vi "DDS_Clock.vi"() -> ()   [LabVIEW 2016] (continued)
  out "frequency-time plot":T6(graph)=[{[{"total time[ms]"=0.0, "f1 [Hz] CH0"=300000000.0}, {"total time[ms]"=0.05, "f1 [Hz] CH0"=300200000.0}, {"total time[ms]"=0.05, "f1 [Hz] CH0"=300200000.0}, {"total time[ms]"=0.1, "f1 [Hz] CH0"=300400000.0}, {"total time[ms]"=0.1, "f1 [Hz] CH0"=300400000.0}, {"total time[ms]"=0.15000000000000002, "f1 [Hz] CH0"=300600000.0}, {"total time[ms]"=0.15000000000000002, "f1 [Hz] CH0"=300600000.0}, {"total time[ms]"=0.2, "f1 [Hz] CH0"=300800000.0}, {"total time[ms]"=0.2, "f1 [Hz] CH0"=300800000.0}, {"total time[ms]"=0.25, "f1 [Hz] CH0"=301000000.0}, {"total time[ms]"=0.25, "f1 [Hz] CH0"=301000000.0}, {"total time[ms]"=0.3, "f1 [Hz] CH0"=301200000.0}, {"total time[ms]"=0.3, "f1 [Hz] CH0"=301200000.0}, {"total time[ms]"=0.35, "f1 [Hz] CH0"=301400000.0}, {"total time[ms]"=0.35, "f1 [Hz] CH0"=301400000.0}, {"total time[ms]"=0.39999999999999997, "f1 [Hz] CH0"=301600000.0}, {"total time[ms]"=0.39999999999999997, "f1 [Hz] CH0"=301600000.0}, {"total time[ms]"=0.44999999999999996, "f1 [Hz] CH0"=301800000.0}, {"total time[ms]"=0.44999999999999996, "f1 [Hz] CH0"=301800000.0}, {"total time[ms]"=0.49999999999999994, "f1 [Hz] CH0"=302000000.0}, {"total time[ms]"=0.49999999999999994, "f1 [Hz] CH0"=302000000.0}, {"total time[ms]"=0.5499999999999999, "f1 [Hz] CH0"=302200000.0}, {"total time[ms]"=0.5499999999999999, "f1 [Hz] CH0"=302200000.0}, {"total time[ms]"=0.6, "f1 [Hz] CH0"=302400000.0}, {"total time[ms]"=0.6, "f1 [Hz] CH0"=302400000.0}, {"total time[ms]"=0.65, "f1 [Hz] CH0"=302600000.0}, {"total time[ms]"=0.65, "f1 [Hz] CH0"=302600000.0}, {"total time[ms]"=0.7000000000000001, "f1 [Hz] CH0"=302800000.0}, {"total time[ms]"=0.7000000000000001, "f1 [Hz] CH0"=302800000.0}, {"total time[ms]"=0.7500000000000001, "f1 [Hz] CH0"=303000000.0}, {"total time[ms]"=0.7500000000000001, "f1 [Hz] CH0"=303000000.0}, {"total time[ms]"=0.8000000000000002, "f1 [Hz] CH0"=303200000.0}, {"total time[ms]"=0.8000000000000002, "f1 [Hz] CH0"=303200000.0}, {"total time[ms]"=0.8500000000000002, "f1 [Hz] CH0"=303400000.0}, {"total time[ms]"=0.8500000000000002, "f1 [Hz] CH0"=303400000.0}, {"total time[ms]"=0.9000000000000002, "f1 [Hz] CH0"=303600000.0}, {"total time[ms]"=0.9000000000000002, "f1 [Hz] CH0"=303600000.0}, {"total time[ms]"=0.9500000000000003, "f1 [Hz] CH0"=303800000.0}, {"total time[ms]"=0.9500000000000003, "f1 [Hz] CH0"=303800000.0}, {"total time[ms]"=1.0000000000000002, "f1 [Hz] CH0"=304000000.0}, {"total time[ms]"=1.0000000000000002, "f1 [Hz] CH0"=304000000.0}, {"total time[ms]"=1.0500000000000003, "f1 [Hz] CH0"=304200000.0}, {"total time[ms]"=1.0500000000000003, "f1 [Hz] CH0"=304200000.0}, {"total time[ms]"=1.1000000000000003, "f1 [Hz] CH0"=304400000.0}, {"total time[ms]"=1.1000000000000003, "f1 [Hz] CH0"=304400000.0}, {"total time[ms]"=1.1500000000000004, "f1 [Hz] CH0"=304600000.0}, {"total time[ms]"=1.1500000000000004, "f1 [Hz] CH0"=304600000.0}, {"total time[ms]"=1.2000000000000004, "f1 [Hz] CH0"=304800000.0}, {"total time[ms]"=1.2000000000000004, "f1 [Hz] CH0"=304800000.0}, {"total time[ms]"=1.2500000000000004, "f1 [Hz] CH0"=305000000.0}, {"total time[ms]"=1.2500000000000004, "f1 [Hz] CH0"=305000000.0}, {"total time[ms]"=1.3000000000000005, "f1 [Hz] CH0"=305200000.0}, {"total time[ms]"=1.3000000000000005, "f1 [Hz] CH0"=305200000.0}, {"total time[ms]"=1.3500000000000005, "f1 [Hz] CH0"=305400000.0}, {"total time[ms]"=1.3500000000000005, "f1 [Hz] CH0"=305400000.0}, {"total time[ms]"=1.4000000000000006, "f1 [Hz] CH0"=305600000.0}, {"total time[ms]"=1.4000000000000006, "f1 [Hz] CH0"=305600000.0}, {"total time[ms]"=1.4500000000000006, "f1 [Hz] CH0"=305800000.0}, {"total time[ms]"=1.4500000000000006, "f1 [Hz] CH0"=305800000.0}, {"total time[ms]"=1.5000000000000007, "f1 [Hz] CH0"=306000000.0}, {"total time[ms]"=1.5000000000000007, "f1 [Hz] CH0"=306000000.0}, {"total time[ms]"=1.5500000000000007, "f1 [Hz] CH0"=306200000.0}, {"total time[ms]"=1.5500000000000007, "f1 [Hz] CH0"=306200000.0}, {"total time[ms]"=1.6000000000000008, "f1 [Hz] CH0"=306400000.0}, {"total time[ms]"=1.6000000000000008, "f1 [Hz] CH0"=306400000.0}, {"total time[ms]"=1.6500000000000008, "f1 [Hz] CH0"=306600000.0}, {"total time[ms]"=1.6500000000000008, "f1 [Hz] CH0"=306600000.0}, {"total time[ms]"=1.7000000000000008, "f1 [Hz] CH0"=306800000.0}, {"total time[ms]"=1.7000000000000008, "f1 [Hz] CH0"=306800000.0}, {"total time[ms]"=1.7500000000000009, "f1 [Hz] CH0"=307000000.0}, {"total time[ms]"=1.7500000000000009, "f1 [Hz] CH0"=307000000.0}, {"total time[ms]"=1.800000000000001, "f1 [Hz] CH0"=307200000.0}, {"total time[ms]"=1.800000000000001, "f1 [Hz] CH0"=307200000.0}, {"total time[ms]"=1.850000000000001, "f1 [Hz] CH0"=307400000.0}, {"total time[ms]"=1.850000000000001, "f1 [Hz] CH0"=307400000.0}, {"total time[ms]"=1.900000000000001, "f1 [Hz] CH0"=307600000.0}, {"total time[ms]"=1.900000000000001, "f1 [Hz] CH0"=307600000.0}, {"total time[ms]"=1.950000000000001, "f1 [Hz] CH0"=307800000.0}, {"total time[ms]"=1.950000000000001, "f1 [Hz] CH0"=307800000.0}, {"total time[ms]"=2.000000000000001, "f1 [Hz] CH0"=308000000.0}, {"total time[ms]"=2.000000000000001, "f1 [Hz] CH0"=308000000.0}, {"total time[ms]"=2.0500000000000007, "f1 [Hz] CH0"=308200000.0}, {"total time[ms]"=2.0500000000000007, "f1 [Hz] CH0"=308200000.0}, {"total time[ms]"=2.1000000000000005, "f1 [Hz] CH0"=308400000.0}, {"total time[ms]"=2.1000000000000005, "f1 [Hz] CH0"=308400000.0}, {"total time[ms]"=2.1500000000000004, "f1 [Hz] CH0"=308600000.0}, {"total time[ms]"=2.1500000000000004, "f1 [Hz] CH0"=308600000.0}, {"total time[ms]"=2.2, "f1 [Hz] CH0"=308800000.0}, {"total time[ms]"=2.2, "f1 [Hz] CH0"=308800000.0}, {"total time[ms]"=2.25, "f1 [Hz] CH0"=309000000.0}, {"total time[ms]"=2.25, "f1 [Hz] CH0"=309000000.0}, {"total time[ms]"=2.3, "f1 [Hz] CH0"=309200000.0}, {"total time[ms]"=2.3, "f1 [Hz] CH0"=309200000.0}, {"total time[ms]"=2.3499999999999996, "f1 [Hz] CH0"=309400000.0}, {"total time[ms]"=2.3499999999999996, "f1 [Hz] CH0"=309400000.0}, {"total time[ms]"=2.3999999999999995, "f1 [Hz] CH0"=309600000.0}, {"total time[ms]"=2.3999999999999995, "f1 [Hz] CH0"=309600000.0}, {"total time[ms]"=2.4499999999999993, "f1 [Hz] CH0"=309800000.0}, {"total time[ms]"=2.4499999999999993, "f1 [Hz] CH0"=309800000.0}, {"total time[ms]"=2.499999999999999, "f1 [Hz] CH0"=310000000.0}, {"total time[ms]"=2.499999999999999, "f1 [Hz] CH0"=310000000.0}, {"total time[ms]"=2.549999999999999, "f1 [Hz] CH0"=310200000.0}, {"total time[ms]"=2.549999999999999, "f1 [Hz] CH0"=310200000.0}, {"total time[ms]"=2.5999999999999988, "f1 [Hz] CH0"=310400000.0}, {"total time[ms]"=2.5999999999999988, "f1 [Hz] CH0"=310400000.0}, {"total time[ms]"=2.6499999999999986, "f1 [Hz] CH0"=310600000.0}, {"total time[ms]"=2.6499999999999986, "f1 [Hz] CH0"=310600000.0}, {"total time[ms]"=2.6999999999999984, "f1 [Hz] CH0"=310800000.0}, {"total time[ms]"=2.6999999999999984, "f1 [Hz] CH0"=310800000.0}, {"total time[ms]"=2.7499999999999982, "f1 [Hz] CH0"=311000000.0}, {"total time[ms]"=2.7499999999999982, "f1 [Hz] CH0"=311000000.0}, {"total time[ms]"=2.799999999999998, "f1 [Hz] CH0"=311200000.0}, {"total time[ms]"=2.799999999999998, "f1 [Hz] CH0"=311200000.0}, {"total time[ms]"=2.849999999999998, "f1 [Hz] CH0"=311400000.0}, {"total time[ms]"=2.849999999999998, "f1 [Hz] CH0"=311400000.0}, {"total time[ms]"=2.8999999999999977, "f1 [Hz] CH0"=311600000.0}, {"total time[ms]"=2.8999999999999977, "f1 [Hz] CH0"=311600000.0}, {"total time[ms]"=2.9499999999999975, "f1 [Hz] CH0"=311800000.0}, {"total time[ms]"=2.9499999999999975, "f1 [Hz] CH0"=311800000.0}, {"total time[ms]"=2.9999999999999973, "f1 [Hz] CH0"=312000000.0}, {"total time[ms]"=2.9999999999999973, "f1 [Hz] CH0"=312000000.0}, {"total time[ms]"=3.049999999999997, "f1 [Hz] CH0"=312200000.0}, {"total time[ms]"=3.049999999999997, "f1 [Hz] CH0"=312200000.0}, {"total time[ms]"=3.099999999999997, "f1 [Hz] CH0"=312400000.0}, {"total time[ms]"=3.099999999999997, "f1 [Hz] CH0"=312400000.0}, {"total time[ms]"=3.149999999999997, "f1 [Hz] CH0"=312600000.0}, {"total time[ms]"=3.149999999999997, "f1 [Hz] CH0"=312600000.0}, {"total time[ms]"=3.1999999999999966, "f1 [Hz] CH0"=312800000.0}, {"total time[ms]"=3.1999999999999966, "f1 [Hz] CH0"=312800000.0}, {"total time[ms]"=3.2499999999999964, "f1 [Hz] CH0"=313000000.0}, {"total time[ms]"=3.2499999999999964, "f1 [Hz] CH0"=313000000.0}, {"total time[ms]"=3.2999999999999963, "f1 [Hz] CH0"=313200000.0}, {"total time[ms]"=3.2999999999999963, "f1 [Hz] CH0"=313200000.0}, {"total time[ms]"=3.349999999999996, "f1 [Hz] CH0"=313400000.0}, {"total time[ms]"=3.349999999999996, "f1 [Hz] CH0"=313400000.0}, {"total time[ms]"=3.399999999999996, "f1 [Hz] CH0"=313600000.0}, {"total time[ms]"=3.399999999999996, "f1 [Hz] CH0"=313600000.0}, {"total time[ms]"=3.4499999999999957, "f1 [Hz] CH0"=313800000.0}, {"total time[ms]"=3.4499999999999957, "f1 [Hz] CH0"=313800000.0}, {"total time[ms]"=3.4999999999999956, "f1 [Hz] CH0"=314000000.0}, {"total time[ms]"=3.4999999999999956, "f1 [Hz] CH0"=314000000.0}, {"total time[ms]"=3.5499999999999954, "f1 [Hz] CH0"=314200000.0}, {"total time[ms]"=3.5499999999999954, "f1 [Hz] CH0"=314200000.0}, {"total time[ms]"=3.599999999999995, "f1 [Hz] CH0"=314400000.0}, {"total time[ms]"=3.599999999999995, "f1 [Hz] CH0"=314400000.0}, {"total time[ms]"=3.649999999999995, "f1 [Hz] CH0"=314600000.0}, {"total time[ms]"=3.649999999999995, "f1 [Hz] CH0"=314600000.0}, {"total time[ms]"=3.699999999999995, "f1 [Hz] CH0"=314800000.0}, {"total time[ms]"=3.699999999999995, "f1 [Hz] CH0"=314800000.0}, {"total time[ms]"=3.7499999999999947, "f1 [Hz] CH0"=315000000.0}, {"total time[ms]"=3.7499999999999947, "f1 [Hz] CH0"=315000000.0}, {"total time[ms]"=3.7999999999999945, "f1 [Hz] CH0"=315200000.0}, {"total time[ms]"=3.7999999999999945, "f1 [Hz] CH0"=315200000.0}, {"total time[ms]"=3.8499999999999943, "f1 [Hz] CH0"=315400000.0}, {"total time[ms]"=3.8499999999999943, "f1 [Hz] CH0"=315400000.0}, {"total time[ms]"=3.899999999999994, "f1 [Hz] CH0"=315600000.0}, {"total time[ms]"=3.899999999999994, "f1 [Hz] CH0"=315600000.0}, {"total time[ms]"=3.949999999999994, "f1 [Hz] CH0"=315800000.0}, {"total time[ms]"=3.949999999999994, "f1 [Hz] CH0"=315800000.0}, {"total time[ms]"=3.999999999999994, "f1 [Hz] CH0"=316000000.0}, {"total time[ms]"=3.999999999999994, "f1 [Hz] CH0"=316000000.0}, {"total time[ms]"=4.049999999999994, "f1 [Hz] CH0"=316200000.0}, {"total time[ms]"=4.049999999999994, "f1 [Hz] CH0"=316200000.0}, {"total time[ms]"=4.099999999999993, "f1 [Hz] CH0"=316400000.0}, {"total time[ms]"=4.099999999999993, "f1 [Hz] CH0"=316400000.0}, {"total time[ms]"=4.149999999999993, "f1 [Hz] CH0"=316600000.0}, {"total time[ms]"=4.149999999999993, "f1 [Hz] CH0"=316600000.0}, {"total time[ms]"=4.199999999999993, "f1 [Hz] CH0"=316800000.0}, {"total time[ms]"=4.199999999999993, "f1 [Hz] CH0"=316800000.0}, {"total time[ms]"=4.249999999999993, "f1 [Hz] CH0"=317000000.0}, {"total time[ms]"=4.249999999999993, "f1 [Hz] CH0"=317000000.0}, {"total time[ms]"=4.299999999999993, "f1 [Hz] CH0"=317200000.0}, {"total time[ms]"=4.299999999999993, "f1 [Hz] CH0"=317200000.0}, {"total time[ms]"=4.3499999999999925, "f1 [Hz] CH0"=317400000.0}, {"total time[ms]"=4.3499999999999925, "f1 [Hz] CH0"=317400000.0}, {"total time[ms]"=4.399999999999992, "f1 [Hz] CH0"=317600000.0}, {"total time[ms]"=4.399999999999992, "f1 [Hz] CH0"=317600000.0}, {"total time[ms]"=4.449999999999992, "f1 [Hz] CH0"=317800000.0}, {"total time[ms]"=4.449999999999992, "f1 [Hz] CH0"=317800000.0}, {"total time[ms]"=4.499999999999992, "f1 [Hz] CH0"=318000000.0}, {"total time[ms]"=4.499999999999992, "f1 [Hz] CH0"=318000000.0}, {"total time[ms]"=4.549999999999992, "f1 [Hz] CH0"=318200000.0}, {"total time[ms]"=4.549999999999992, "f1 [Hz] CH0"=318200000.0}, {"total time[ms]"=4.599999999999992, "f1 [Hz] CH0"=318400000.0}, {"total time[ms]"=4.599999999999992, "f1 [Hz] CH0"=318400000.0}, {"total time[ms]"=4.6499999999999915, "f1 [Hz] CH0"=318600000.0}, {"total time[ms]"=4.6499999999999915, "f1 [Hz] CH0"=318600000.0}, {"total time[ms]"=4.699999999999991, "f1 [Hz] CH0"=318800000.0}, {"total time[ms]"=4.699999999999991, "f1 [Hz] CH0"=318800000.0}, {"total time[ms]"=4.749999999999991, "f1 [Hz] CH0"=319000000.0}, {"total time[ms]"=4.749999999999991, "f1 [Hz] CH0"=319000000.0}, {"total time[ms]"=4.799999999999991, "f1 [Hz] CH0"=319200000.0}, {"total time[ms]"=4.799999999999991, "f1 [Hz] CH0"=319200000.0}, {"total time[ms]"=4.849999999999991, "f1 [Hz] CH0"=319400000.0}, {"total time[ms]"=4.849999999999991, "f1 [Hz] CH0"=319400000.0}, {"total time[ms]"=4.899999999999991, "f1 [Hz] CH0"=319600000.0}, {"total time[ms]"=4.899999999999991, "f1 [Hz] CH0"=319600000.0}, {"total time[ms]"=4.94999999999999, "f1 [Hz] CH0"=319800000.0}, {"total time[ms]"=4.94999999999999, "f1 [Hz] CH0"=319800000.0}, {"total time[ms]"=4.99999999999999, "f1 [Hz] CH0"=320000000.0}, {"total time[ms]"=4.99999999999999, "f1 [Hz] CH0"=320000000.0}, {"total time[ms]"=5.04999999999999, "f1 [Hz] CH0"=319800000.0}, {"total time[ms]"=5.04999999999999, "f1 [Hz] CH0"=319800000.0}, {"total time[ms]"=5.09999999999999, "f1 [Hz] CH0"=319600000.0}, {"total time[ms]"=5.09999999999999, "f1 [Hz] CH0"=319600000.0}, {"total time[ms]"=5.14999999999999, "f1 [Hz] CH0"=319400000.0}, {"total time[ms]"=5.14999999999999, "f1 [Hz] CH0"=319400000.0}, {"total time[ms]"=5.1999999999999895, "f1 [Hz] CH0"=319200000.0}, {"total time[ms]"=5.1999999999999895, "f1 [Hz] CH0"=319200000.0}, {"total time[ms]"=5.249999999999989, "f1 [Hz] CH0"=319000000.0}, {"total time[ms]"=5.249999999999989, "f1 [Hz] CH0"=319000000.0}, {"total time[ms]"=5.299999999999989, "f1 [Hz] CH0"=318800000.0}, {"total time[ms]"=5.299999999999989, "f1 [Hz] CH0"=318800000.0}, {"total time[ms]"=5.349999999999989, "f1 [Hz] CH0"=318600000.0}, {"total time[ms]"=5.349999999999989, "f1 [Hz] CH0"=318600000.0}, {"total time[ms]"=5.399999999999989, "f1 [Hz] CH0"=318400000.0}, {"total time[ms]"=5.399999999999989, "f1 [Hz] CH0"=318400000.0}, {"total time[ms]"=5.449999999999989, "f1 [Hz] CH0"=318200000.0}, {"total time[ms]"=5.449999999999989, "f1 [Hz] CH0"=318200000.0}, {"total time[ms]"=5.4999999999999885, "f1 [Hz] CH0"=318000000.0}, {"total time[ms]"=5.4999999999999885, "f1 [Hz] CH0"=318000000.0}, {"total time[ms]"=5.549999999999988, "f1 [Hz] CH0"=317800000.0}, {"total time[ms]"=5.549999999999988, "f1 [Hz] CH0"=317800000.0}, {"total time[ms]"=5.599999999999988, "f1 [Hz] CH0"=317600000.0}, {"total time[ms]"=5.599999999999988, "f1 [Hz] CH0"=317600000.0}, {"total time[ms]"=5.649999999999988, "f1 [Hz] CH0"=317400000.0}, {"total time[ms]"=5.649999999999988, "f1 [Hz] CH0"=317400000.0}, {"total time[ms]"=5.699999999999988, "f1 [Hz] CH0"=317200000.0}, {"total time[ms]"=5.699999999999988, "f1 [Hz] CH0"=317200000.0}, {"total time[ms]"=5.749999999999988, "f1 [Hz] CH0"=317000000.0}, {"total time[ms]"=5.749999999999988, "f1 [Hz] CH0"=317000000.0}, {"total time[ms]"=5.799999999999987, "f1 [Hz] CH0"=316800000.0}, {"total time[ms]"=5.799999999999987, "f1 [Hz] CH0"=316800000.0}, {"total time[ms]"=5.849999999999987, "f1 [Hz] CH0"=316600000.0}, {"total time[ms]"=5.849999999999987, "f1 [Hz] CH0"=316600000.0}, {"total time[ms]"=5.899999999999987, "f1 [Hz] CH0"=316400000.0}, {"total time[ms]"=5.899999999999987, "f1 [Hz] CH0"=316400000.0}, {"total time[ms]"=5.949999999999987, "f1 [Hz] CH0"=316200000.0}, {"total time[ms]"=5.949999999999987, "f1 [Hz] CH0"=316200000.0}, {"total time[ms]"=5.999999999999987, "f1 [Hz] CH0"=316000000.0}, {"total time[ms]"=5.999999999999987, "f1 [Hz] CH0"=316000000.0}, {"total time[ms]"=6.0499999999999865, "f1 [Hz] CH0"=315800000.0}, {"total time[ms]"=6.0499999999999865, "f1 [Hz] CH0"=315800000.0}, {"total time[ms]"=6.099999999999986, "f1 [Hz] CH0"=315600000.0}, {"total time[ms]"=6.099999999999986, "f1 [Hz] CH0"=315600000.0}, {"total time[ms]"=6.149999999999986, "f1 [Hz] CH0"=315400000.0}, {"total time[ms]"=6.149999999999986, "f1 [Hz] CH0"=315400000.0}, {"total time[ms]"=6.199999999999986, "f1 [Hz] CH0"=315200000.0}, {"total time[ms]"=6.199999999999986, "f1 [Hz] CH0"=315200000.0}, {"total time[ms]"=6.249999999999986, "f1 [Hz] CH0"=315000000.0}, {"total time[ms]"=6.249999999999986, "f1 [Hz] CH0"=315000000.0}, {"total time[ms]"=6.299999999999986, "f1 [Hz] CH0"=314800000.0}, {"total time[ms]"=6.299999999999986, "f1 [Hz] CH0"=314800000.0}, {"total time[ms]"=6.349999999999985, "f1 [Hz] CH0"=314600000.0}, {"total time[ms]"=6.349999999999985, "f1 [Hz] CH0"=314600000.0}, {"total time[ms]"=6.399999999999985, "f1 [Hz] CH0"=314400000.0}, {"total time[ms]"=6.399999999999985, "f1 [Hz] CH0"=314400000.0}, {"total time[ms]"=6.449999999999985, "f1 [Hz] CH0"=314200000.0}, {"total time[ms]"=6.449999999999985, "f1 [Hz] CH0"=314200000.0}, {"total time[ms]"=6.499999999999985, "f1 [Hz] CH0"=314000000.0}, {"total time[ms]"=6.499999999999985, "f1 [Hz] CH0"=314000000.0}, {"total time[ms]"=6.549999999999985, "f1 [Hz] CH0"=313800000.0}, {"total time[ms]"=6.549999999999985, "f1 [Hz] CH0"=313800000.0}, {"total time[ms]"=6.5999999999999845, "f1 [Hz] CH0"=313600000.0}, {"total time[ms]"=6.5999999999999845, "f1 [Hz] CH0"=313600000.0}, {"total time[ms]"=6.649999999999984, "f1 [Hz] CH0"=313400000.0}, {"total time[ms]"=6.649999999999984, "f1 [Hz] CH0"=313400000.0}, {"total time[ms]"=6.699999999999984, "f1 [Hz] CH0"=313200000.0}, {"total time[ms]"=6.699999999999984, "f1 [Hz] CH0"=313200000.0}, {"total time[ms]"=6.749999999999984, "f1 [Hz] CH0"=313000000.0}, {"total time[ms]"=6.749999999999984, "f1 [Hz] CH0"=313000000.0}, {"total time[ms]"=6.799999999999984, "f1 [Hz] CH0"=312800000.0}, {"total time[ms]"=6.799999999999984, "f1 [Hz] CH0"=312800000.0}, {"total time[ms]"=6.849999999999984, "f1 [Hz] CH0"=312600000.0}, {"total time[ms]"=6.849999999999984, "f1 [Hz] CH0"=312600000.0}, {"total time[ms]"=6.8999999999999835, "f1 [Hz] CH0"=312400000.0}, {"total time[ms]"=6.8999999999999835, "f1 [Hz] CH0"=312400000.0}, {"total time[ms]"=6.949999999999983, "f1 [Hz] CH0"=312200000.0}, {"total time[ms]"=6.949999999999983, "f1 [Hz] CH0"=312200000.0}, {"total time[ms]"=6.999999999999983, "f1 [Hz] CH0"=312000000.0}, {"total time[ms]"=6.999999999999983, "f1 [Hz] CH0"=312000000.0}, {"total time[ms]"=7.049999999999983, "f1 [Hz] CH0"=311800000.0}, {"total time[ms]"=7.049999999999983, "f1 [Hz] CH0"=311800000.0}, {"total time[ms]"=7.099999999999983, "f1 [Hz] CH0"=311600000.0}, {"total time[ms]"=7.099999999999983, "f1 [Hz] CH0"=311600000.0}, {"total time[ms]"=7.149999999999983, "f1 [Hz] CH0"=311400000.0}, {"total time[ms]"=7.149999999999983, "f1 [Hz] CH0"=311400000.0}, {"total time[ms]"=7.199999999999982, "f1 [Hz] CH0"=311200000.0}, {"total time[ms]"=7.199999999999982, "f1 [Hz] CH0"=311200000.0}, {"total time[ms]"=7.249999999999982, "f1 [Hz] CH0"=311000000.0}, {"total time[ms]"=7.249999999999982, "f1 [Hz] CH0"=311000000.0}, {"total time[ms]"=7.299999999999982, "f1 [Hz] CH0"=310800000.0}, {"total time[ms]"=7.299999999999982, "f1 [Hz] CH0"=310800000.0}, {"total time[ms]"=7.349999999999982, "f1 [Hz] CH0"=310600000.0}, {"total time[ms]"=7.349999999999982, "f1 [Hz] CH0"=310600000.0}, {"total time[ms]"=7.399999999999982, "f1 [Hz] CH0"=310400000.0}, {"total time[ms]"=7.399999999999982, "f1 [Hz] CH0"=310400000.0}, {"total time[ms]"=7.4499999999999815, "f1 [Hz] CH0"=310200000.0}, {"total time[ms]"=7.4499999999999815, "f1 [Hz] CH0"=310200000.0}, {"total time[ms]"=7.499999999999981, "f1 [Hz] CH0"=310000000.0}, {"total time[ms]"=7.499999999999981, "f1 [Hz] CH0"=310000000.0}, {"total time[ms]"=7.549999999999981, "f1 [Hz] CH0"=309800000.0}, {"total time[ms]"=7.549999999999981, "f1 [Hz] CH0"=309800000.0}, {"total time[ms]"=7.599999999999981, "f1 [Hz] CH0"=309600000.0}, {"total time[ms]"=7.599999999999981, "f1 [Hz] CH0"=309600000.0}, {"total time[ms]"=7.649999999999981, "f1 [Hz] CH0"=309400000.0}, {"total time[ms]"=7.649999999999981, "f1 [Hz] CH0"=309400000.0}, {"total time[ms]"=7.699999999999981, "f1 [Hz] CH0"=309200000.0}, {"total time[ms]"=7.699999999999981, "f1 [Hz] CH0"=309200000.0}, {"total time[ms]"=7.7499999999999805, "f1 [Hz] CH0"=309000000.0}, {"total 
